vi "Insert Mission Logo.vi"(8 "error in":errorcluster, 11 "Test Selector in":refnum<class "Test Selector.lvclass">) -> (0 "error out":errorcluster, 3 "Test Selector out":refnum<class "Test Selector.lvclass">)   [LabVIEW 2019, in "Test Selector.lvlib" / "Test Selector.lvclass"]
uses:
  Test Selector.lvclass
  Test Selector.lvclass/Test Selector.ctl
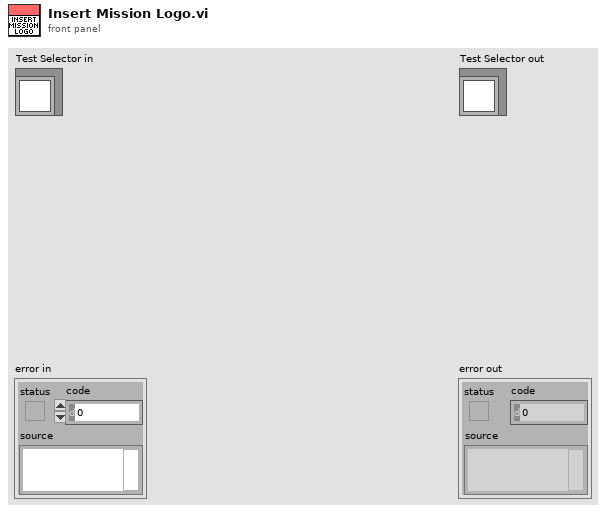
[diagram p1: front panel]
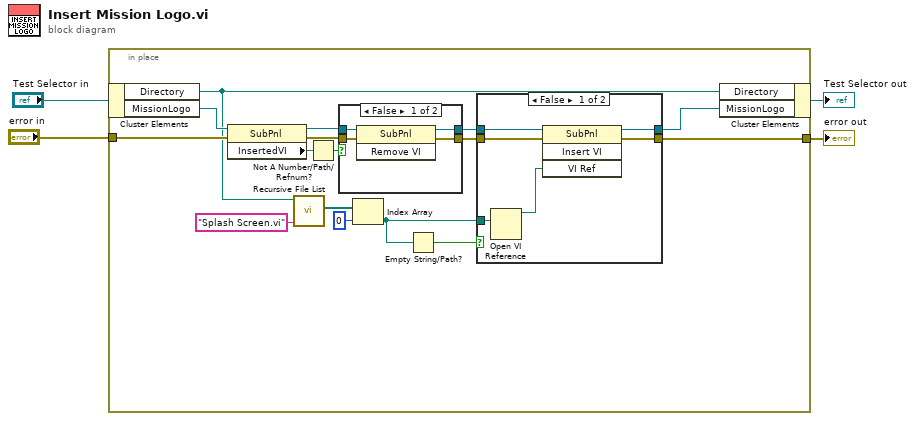
[diagram p0: block diagram]
diagram:
  n1 = in-place {
    in-place-border: "error in" -> [w7]
    in-place-border: [w6] -> w1
    n2 = in-place-cluster #1("Test Selector in") -> ("Directory"=w5:path, "MissionLogo"=w20:refnum<vi>)
    n3 = property class="SubPnl"(reference=w20, error in=w7) -> (reference out=w19:refnum<vi>, error out=w18:errorcluster, "InsertedVI"=w17:refnum<vi>)
    n4 = call <vilib>:"Recursive File List.vi"("pattern"="Splash Screen.vi" ("name or relative path"), "Folder Path"=w5) -> ("All Files in Dir"=w11:path[])  [unwired: 5 in, 4 out]
    n5 = Not A Number/Path/Refnum?(number/path/refnum=w17) -> (NaN/Path/Refnum?=w16:bool)
    n6 = case shown="False" w16 {
      tunnel: w19 -> [w32 w34]
      tunnel: [w31 w34] -> w15
      tunnel: w18 -> [w30 w33]
      tunnel: [w29 w33] -> w13
      frame False {
        n7 = invoke class="SubPnl" method="Remove VI"(reference=w32, error in=w30) -> (reference out=w31:refnum<vi>, error out=w29:errorcluster)  [unwired: 1 in, 1 out]
      }
      frame True {
      }
    }
    n8 = Index Array(array=w11, index=0) -> (element=w8:path)
    n9 = Empty String/Path?(string/path=w8) -> (empty?=w9:bool)
    n10 = case shown="False" w9 {
      tunnel: w15 -> [w26 w27]
      tunnel: w13 -> [w24 w28]
      tunnel: [w23 w28] -> w6
      tunnel: w8 -> [w22 _]
      tunnel: [w21 w27] -> w14
      frame False {
        n11 = Open VI Reference(vi path=w22) -> (vi reference=w25:refnum<vi>)  [unwired: 5 in, 1 out]
        n12 = invoke class="SubPnl" method="Insert VI"(reference=w26, error in=w24, "VI Ref"=w25) -> (reference out=w21:refnum<vi>, error out=w23:errorcluster)  [unwired: 1 in, 2 out]
      }
      frame True {
      }
    }
    n13 = in-place-cluster #1("Directory"=w5, "MissionLogo"=w14) -> (→"Test Selector out":refnum<class "Test Selector.lvclass">)
  }
  "error out" <- w1
